vi "terminate.vi"(8 "error in (no error)":errorcluster, 11 "GenericPlugin in":refnum<class "SignalWriterDL101123SoundCard.lvclass">) -> (0 "error out":errorcluster, 3 "GenericPlugin out":refnum<class "SignalWriterDL101123SoundCard.lvclass">)   [LabVIEW 2010, in "SignalWriterDL101123SoundCard.lvclass"]
doc: "The dynamic dispatch version of this VI terminates the plug-in object by releasing all of its resources."
uses:
  SignalWriterDL101123SoundCard.lvclass
  SignalWriterDL101123SoundCard.lvclass/SignalWriterDL101123SoundCard.ctl
  <vilib>/sound2/lvsound2.llb/Sound Output Task ID.ctl
  GenericSignalWriter/GenericSignalWriter/GenericSignalWriter.lvclass
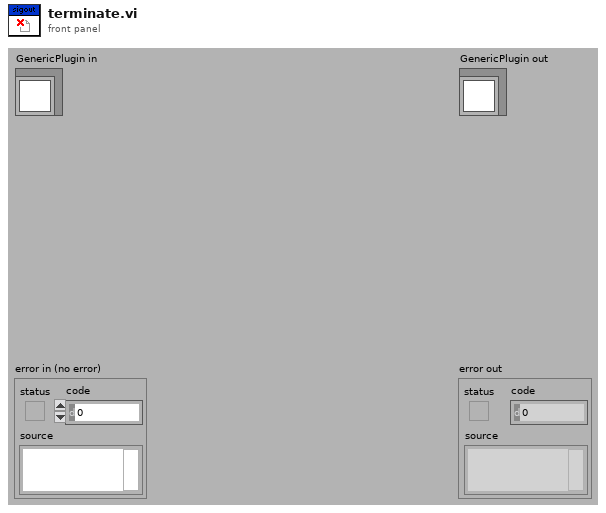
[diagram p1: front panel]
types:
  T1 = typedef "Sound Output Task ID.ctl" = u32
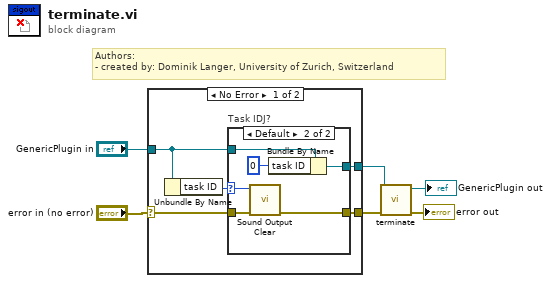
[diagram p0: block diagram]
diagram:
  # "Authors: \n- created by: Dominik Langer, University of Zurich, Switzerland"
  n1 = case shown="No Error" "error in (no error)" {
    selector: "error in (no error)" -> [w11 w20]
    tunnel: [w8 w20] -> w3
    tunnel: "GenericPlugin in" -> [w9 w21]
    tunnel: [w7 w21] -> w1
    frame No Error {
      n2 = Unbundle By Name(w9) -> ("task ID"=w10:T1)
      n3 = case "Task IDJ?" shown="Default" w10 {
        selector: w10 -> [_ w17]
        tunnel: w11 -> [w13 w19]
        tunnel: w9 -> [w12 w16]
        tunnel: [w13 w18] -> w8
        tunnel: [w12 w14] -> w7
        frame 0 {
        }
        frame Default {
          n4 = call <vilib>:"Sound Output Clear.vi"("error in (no error)"=w19, "task ID"=w17) -> ("error out"=w18:errorcluster)  [unwired: 9 in]
          n5 = Bundle By Name(cluster=w16, "task ID"=T1 0) -> (w14:refnum<class "SignalWriterDL101123SoundCard.lvclass">)
        }
      }
    }
    frame Error {
    }
  }
  n6 = call-parent "terminate.vi"("error in (no error)"=w3, "GenericPlugin in"=w1) -> ("error out"=→"error out":errorcluster, "GenericPlugin out"=→"GenericPlugin out":refnum<class "SignalWriterDL101123SoundCard.lvclass">)  [unwired: 8 in]
